vi "0MQ_Server.TestPublisher.vi"() -> ()   [LabVIEW 2016, in "0MQ_Server.lvclass"]
uses:
  0MQ_Server.lvclass
  <vilib>/JKI/JKI SMO/SMO/Typedefs/SMOState --Enum.ctl
  C:/Program Files (x86)/National Instruments/LabVIEW 2016/vi.lib/JKI/JKI SMO/SMO/SMO.lvclass
  Typedefs/Socket Config.ctl
  <vilib>/addons/zeromq/socket_type.ctl
  0MQ_Server.lvclass/0MQ_Server.ctl
  <vilib>/JKI/JKI SMO/SMO/SMO.lvclass
  <vilib>/addons/zeromq/zeromq.lvlib
panel:
  in  "Send":bool
  in  "Message":string
  out "SMO State":T1
  out "error out":errorcluster
  in  "Stop":bool
  # "SMO Test Publisher"
  # "For instructions on how to use the JKI State Machine Objects, examples and video tutorials, visit:\nhttp://jki.net/state-machine-objects/\n\nJKI State Machine Objects™\nhttp://jki.net/state-machine-objects/\nCopyright (C) 2005-2015, JKI <info@jki.net>\nALL RIGHTS RESERVED"
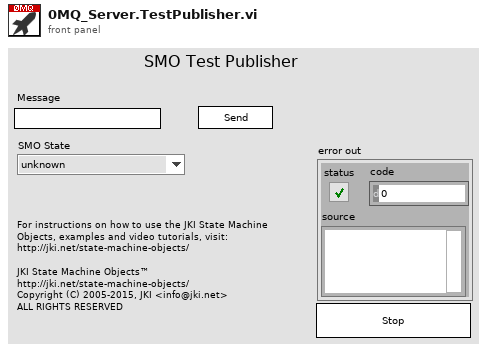
[diagram p1: front panel]
types:
  T1 = typedef "SMO.lvclass/SMOState --Enum.ctl" = enum16{"unknown", "Created", "Started", "Stopped"}
  T2 = typedef "0MQ_Server.lvclass/Socket Config.ctl" = cluster{"Socket type":T3, "endpoint":string, "socket filter":string}
  T3 = typedef "zeromq.lvlib/socket_type.ctl" = enum8{"ZMQ_PAIR", "ZMQ_PUB", "ZMQ_SUB", "ZMQ_REQ", "ZMQ_REP", "ZMQ_DEALER", "ZMQ_ROUTER", "ZMQ_PULL", "ZMQ_PUSH", "ZMQ_XPUB", "ZMQ_XSUB"}
  T4 = typedef "SMO.lvclass/Public Events.ctl" = cluster{"Error":refnum<user-event>, "State":refnum<user-event>, "Reserve State":refnum<user-event>}
  T5 = cluster{"Event Registration Refnum":refnum<event-registration>}
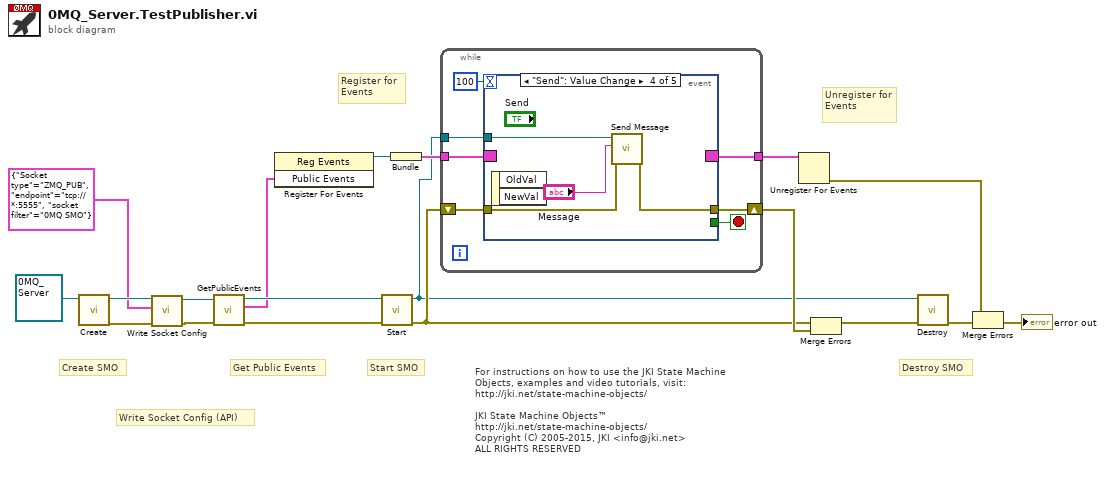
[diagram p0: block diagram]
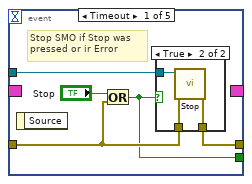
[diagram p2: hidden frame]
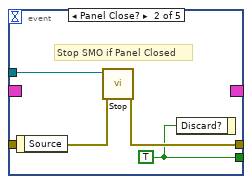
[diagram p4: hidden frame]
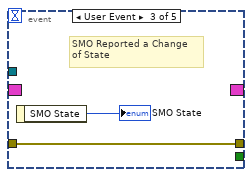
[diagram p5: hidden frame]
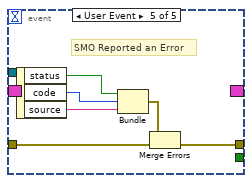
[diagram p6: hidden frame]
diagram:
  # "Write Socket Config (API)"
  # "For instructions on how to use the JKI State Machine Objects, examples and video tutorials, visit:\nhttp://jki.net/state-machine-objects/\n\nJKI State Machine Objects™\nhttp://jki.net/state-machine-objects/\nCopyright (C) 2005-2015, JKI <info@jki.net>\nALL RIGHTS RESERVED"
  # "Get Public Events"
  # "Start SMO"
  # "Destroy SMO"
  # "Create SMO"
  # "Unregister for Events"
  # "Register for Events"
  n1 = call <vilib>:"Create.vi"("SMO"=refnum<class "0MQ_Server.lvclass"> refnum ("SMO.Template.lvclass")) -> ("error out"=w3:errorcluster, "SMO out"=w6:refnum<class "0MQ_Server.lvclass">)  [unwired: 8 in, 1 out]
  n2 = call "Write Socket Config.vi"("error in (no error)"=w3, "Socket Config"=T2 {"Socket type"=enum."ZMQ_PUB", "endpoint"="tcp://*:5555", "socket filter"="0MQ SMO"}, "0MQ_Server in"=w6) -> ("error out"=w4:errorcluster, "0MQ_Server out"=w5:refnum<class "0MQ_Server.lvclass">)  [unwired: 7 in]
  n3 = call <vilib>:"GetPublicEvents.vi"("error in (no error)"=w4, "SMO"=w5) -> ("error out"=w10:errorcluster, "Public Events"=w8:T4, "SMO out"=w9:refnum<class "0MQ_Server.lvclass">)  [unwired: 7 in]
  n4 = register-events(w8) -> (reference out=w7:refnum<event-registration>)  [unwired: 2 in, 1 out]
  n5 = call <vilib>:"Start.vi"("error in (no error)"=w10, "SMO"=w9) -> ("error out"=w12:errorcluster, "SMO out"=w1:refnum<class "0MQ_Server.lvclass">)  [unwired: 8 in]
  n6 = Bundle("Event Registration Refnum"=w7) -> (w18:T5)  [unwired: 1 in]
  n7 = while {
    shift-right: [w25] -> w17
    shift-left: w12 -> [w24]
    tunnel: w18 -> [w23]
    tunnel: [w22] -> w19
    tunnel: w1 -> [w21]
    stop <- w26 stop-if-true
    n8 = event shown="[3] \"Send\": Value Change" {
      selector: w23 -> [_ _ _ _ _]
      dyn-events: [_ _ _ _ _] -> w22
      timeout: 100 -> [_ _ _ _ _]
      tunnel: [w27 w36 _ _ _] -> w26
      tunnel: w21 -> [w31 w39 _ w45 _]
      tunnel: [w30 w38 w41 w42 w47] -> w25
      tunnel: w24 -> [w29 w37 w41 w43 w48]
      event Timeout {
        # "Stop SMO if Stop was \npressed or ir Error"
        n9 = event-data() -> ()  [unwired: 1 in, 1 out]
        n10 = Or(x="Stop", y=w29) -> (x .or. y?=w27:bool)
        n11 = case shown="True" w27 {
          tunnel: w31 -> [_ w35]
          tunnel: [w32 w34] -> w30
          tunnel: w29 -> [w32 w33]
          frame False {
          }
          frame True {
            n12 = call <vilib>:"Stop.vi"("error in (no error)"=w33, "SMO"=w35) -> ("error out"=w34:errorcluster)  [unwired: 8 in, 1 out]
          }
        }
      }
      event Panel Close? {
        w36 = TRUE ("OK")
        # "Stop SMO if Panel Closed"
        n13 = event-data() -> ()  [unwired: 1 in, 1 out]
        n14 = call <vilib>:"Stop.vi"("error in (no error)"=w37, "SMO"=w39) -> ("error out"=w38:errorcluster)  [unwired: 8 in, 1 out]
        n15 = event-data("Discard?"=w36) -> ()  [unwired: 1 in, 1 out]
      }
      event User Event {
        # "SMO Reported a Change\nof State"
        n16 = event-data() -> ("SMO State"=→"SMO State":T1)  [unwired: 1 in]
      }
      event "Send": Value Change {
        n17 = event-data() -> ()  [unwired: 1 in, 2 out]
        n18 = call-dynamic "Send Message.vi"("error in (no error)"=w43, "Message"="Message", "0MQ_Server in"=w45) -> ("error out"=w42:errorcluster)  [unwired: 5 in, 3 out]
      }
      event User Event {
        # "SMO Reported an Error"
        n19 = event-data() -> ("status"=w46:bool, "code"=w50:i32, "source"=w49:string)  [unwired: 1 in]
        n20 = Bundle("status"=w46, "code"=w50, "source"=w49) -> (w51:errorcluster)  [unwired: 1 in]
        n21 = Merge Errors(w51, w48) -> (w47:errorcluster)
      }
    }
  }
  n22 = Unregister For Events(event registration refnum=w19) -> (error out=w16:errorcluster)  [unwired: 1 in]
  n23 = Merge Errors(w12, w17) -> (w11:errorcluster)
  n24 = call <vilib>:"Destroy.vi"("error in (no error)"=w11, "SMO"=w1) -> ("error out"=w14:errorcluster)  [unwired: 9 in]
  n25 = Merge Errors(w16, w14) -> (→"error out":errorcluster)
